vi "Test1_1b_ASIC_pepe.vi"(0 "Instrument VISA in":T1={"AWG VISA"="generadorpulsos", "Oscilloscope  VISA "="Oscilloscope", "Integration Board IP"="172.16.7.43", "connection ID"=refnum, "report out"=refnum, "report file path"=path "D:/CTA/Data_test/ASIC/test3a"}, 1 "threshold":i32[][](array[numeric]), 5 "quantity":i32=3, 7 "Cycles Burst":i32=10000, 11 "error in":errorcluster={"status"=FALSE, "code"=0, "source"="VISA Write in Test2_3a_ASIC_fast.vi->test_sum_ASIC.vi"}, 12 "channel array":i32[](array[numeric])=[0, 1, 2, 3, 4, 5, 6], 13 "Voltages comprobation":dbl[](array[numeric])=[0.05, 0.1, 0.2, 0.3, 0.4, 0.5, 0.6, 0.7, 0.8, 1.0]) -> (4 "Instrument VISA out":T1, 15 "error out":errorcluster)   [LabVIEW 2009]
uses:
  <vilib>/Utility/NIReport.llb/NI_report.lvclass
  <vilib>/Utility/NIReport.llb/HTML/NI_HTML.lvclass
  <instrlib>/Agilent 8000 Series/Public/Configure/Configure Math (Binary Operation).vi
  <instrlib>/Agilent 81150/Agilent 81150.lvlib
  L0_Asic/L0 Asic Test Folder v9/C/Program Files/National Instruments/LabVIEW 2012/instr.lib/Agilent 8000 Series/Agilent 8000 Series.lvlib
panel:
  out "read buffer 4":string="V amptd(f2),1.074E+00,0,1.056E+00,1.087E+00,1.0690E+00,5.5E-03,9.4E+01,+ width(f2),2.90015E-09,0,2.90015E-09,2.95960E-09,2.925838E-09,1.2702E-11,9.4E+01,V amptd(1),5.5E-02,0,4.8E-02,6.7E-02,5.55E-02,3.5E-03,9.4E+01,+ width(f1),9.99999E+37,5,9.99999E+37,9.99999E+37,9.99999E+37,9.99999E+37,9.99999E+37,Time(f1-f2),6.26722E-09,0,6.20145E-09,6.35270E-09,6.264189E-09,3.2805E-11,9.4E+01\n"
  out "report file path":path=path "D:/CTA/Data_test/test3a"
  out "Array":i32[](array[numeric])=[2, 3, 5]
  out "points quantity":dbl=94.0
  out "ouput data array":dbl[](array[numeric])=[0.75, 42.0, 0.0, 63.0, 1.0, 1.069, 0.0055, 2.925838e-09, 1.2702e-11, 0.0555, 0.0035, 9.99999e+37, 9.99999e+37, 6.264189e-09, 3.2805e-11, 94.0]
  out "read buffer 3":string="V amptd(f2),1.074E+00,0,1.056E+00,1.087E+00,1.0690E+00,5.5E-03,9.4E+01,+ width(f2),2.90015E-09,0,2.90015E-09,2.95960E-09,2.925838E-09,1.2702E-11,9.4E+01,V amptd(1),5.5E-02,0,4.8E-02,6.7E-02,5.55E-02,3.5E-03,9.4E+01,+ width(f1),9.99999E+37,5,9.99999E+37,9.99999E+37,9.99999E+37,9.99999E+37,9.99999E+37,Time(f1-f2),6.26722E-09,0,6.20145E-09,6.35270E-09,6.264189E-09,3.2805E-11,9.4E+01\n"
  in  "Voltage":dbl[](array[numeric])=[0.05, 0.2, 0.5, 0.7, 1.0]
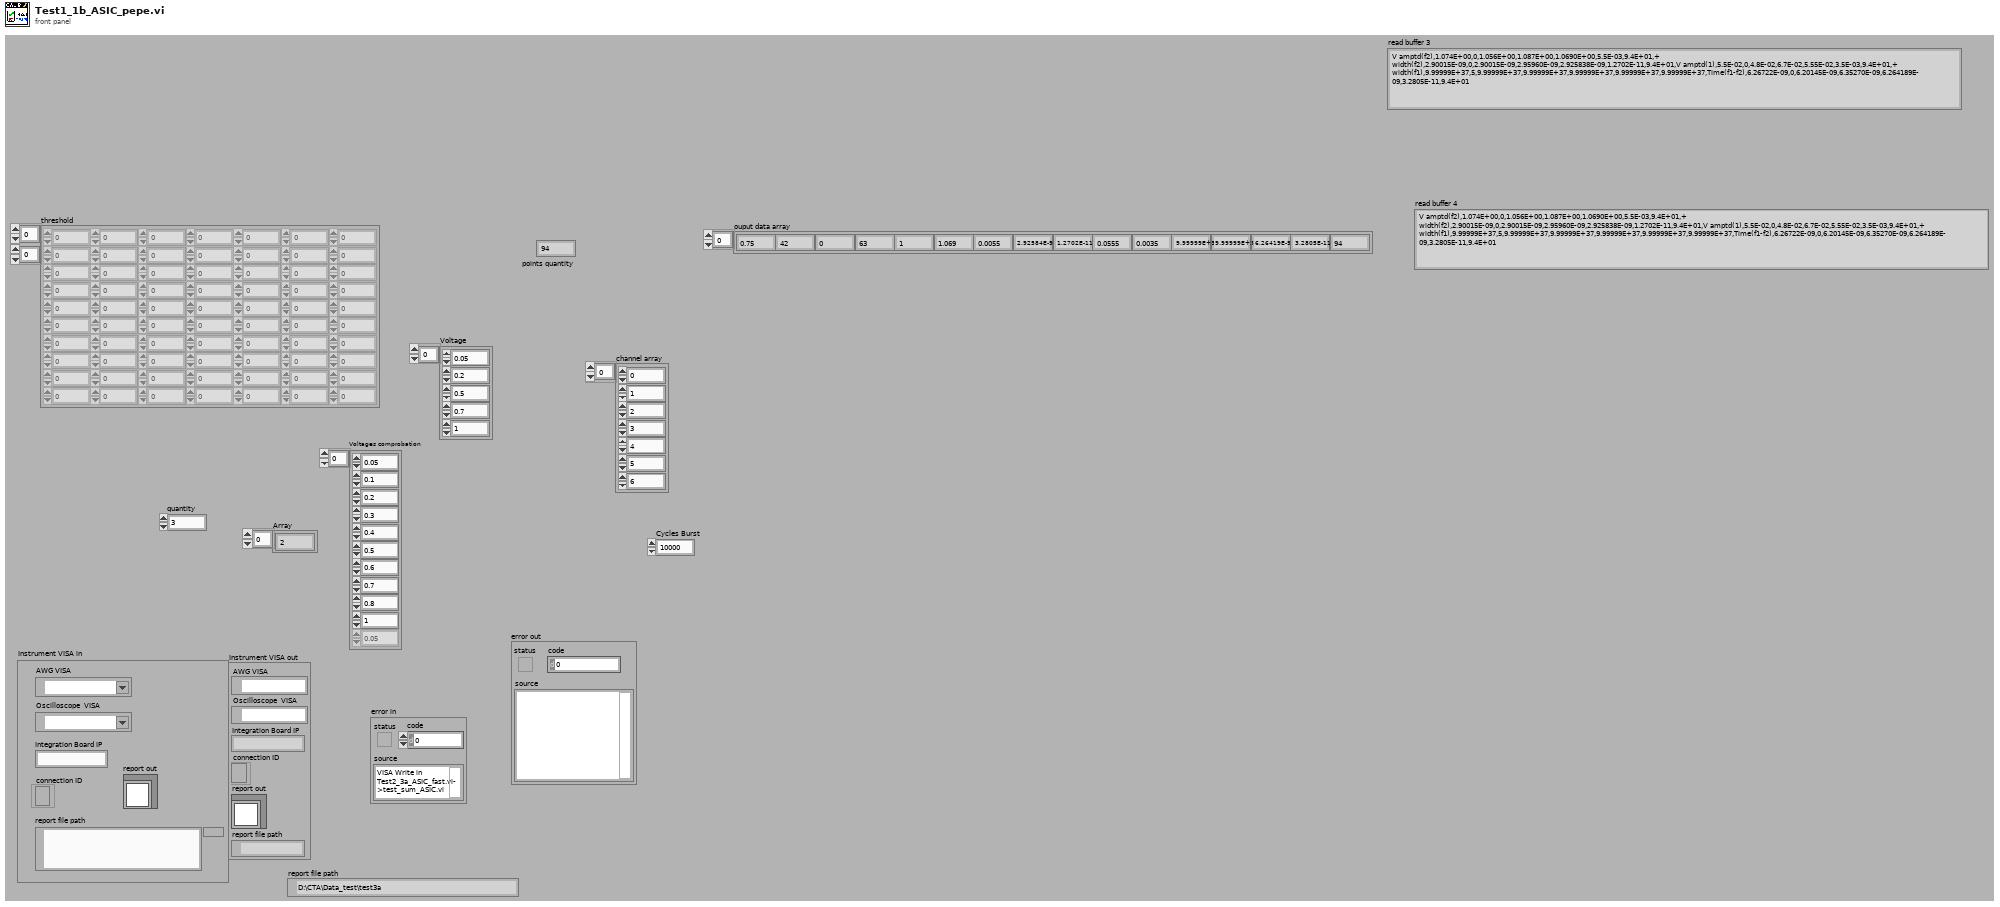
[diagram p1: front panel]
types:
  T1 = cluster{"AWG VISA":refnum<visa-resource-name>, "Oscilloscope  VISA ":refnum<visa-resource-name>, "Integration Board IP":string, "connection ID":refnum<k5>, "report out":refnum<class "NI_report.lvclass">, "report file path":path}
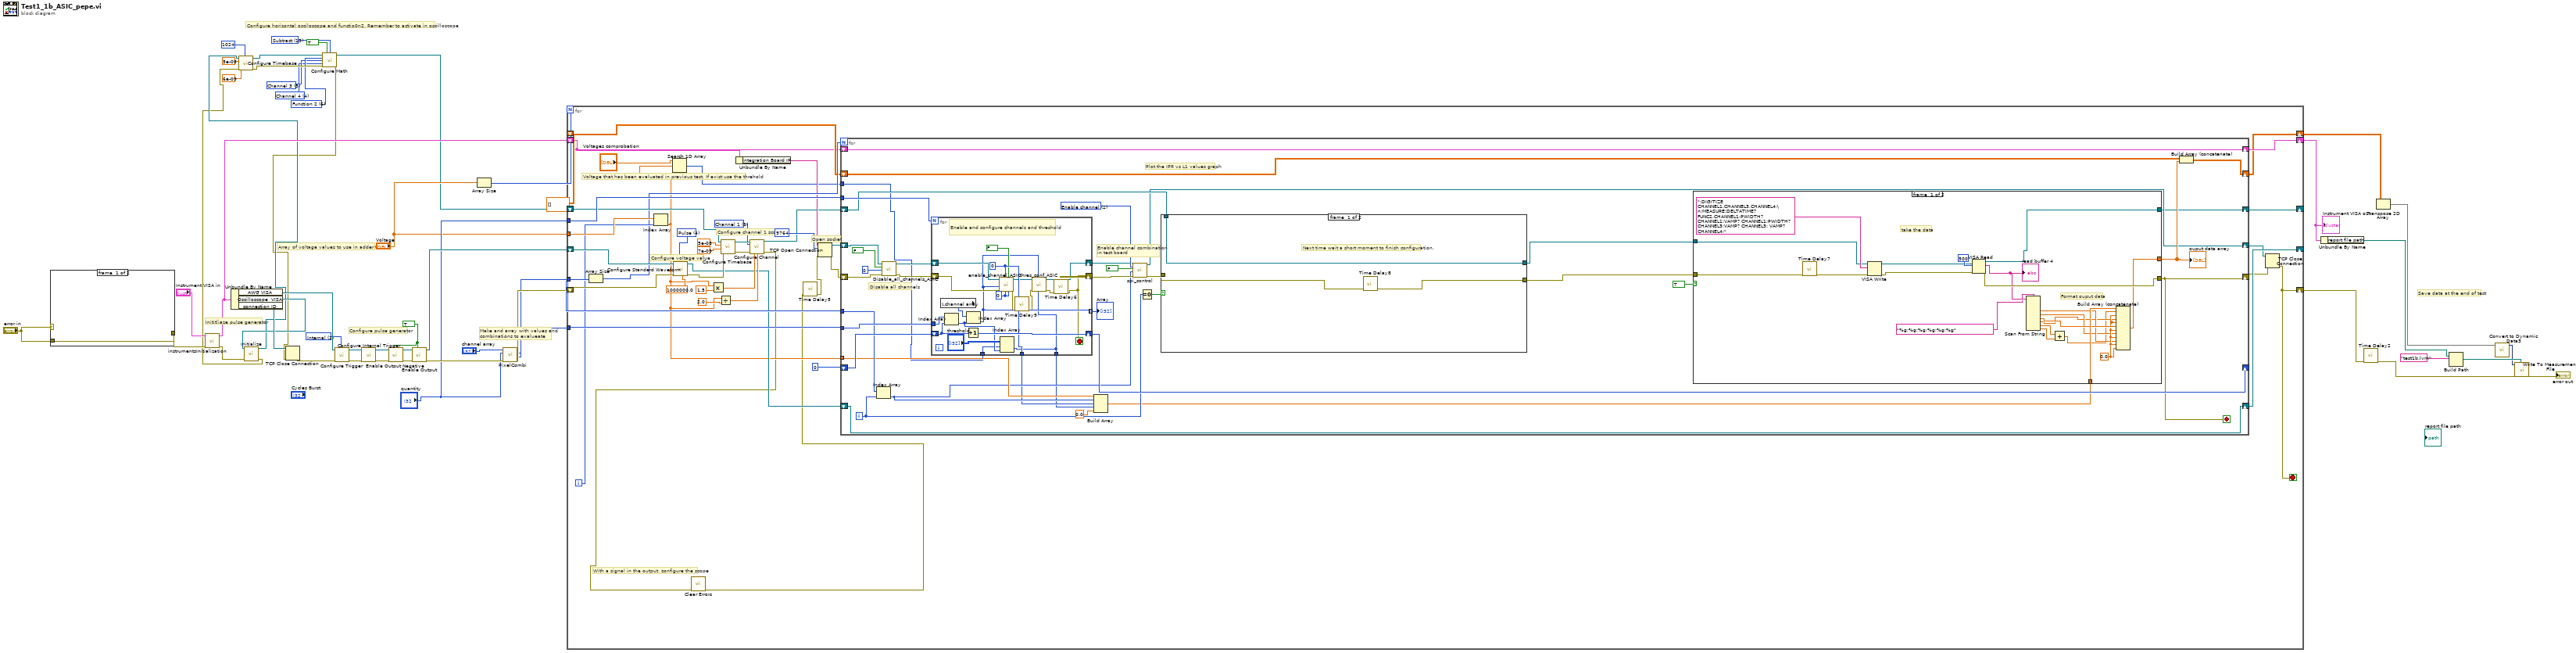
[diagram p0: block diagram]
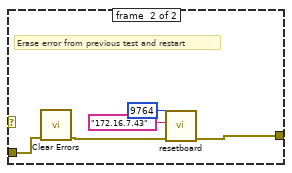
[diagram p2: hidden frame]
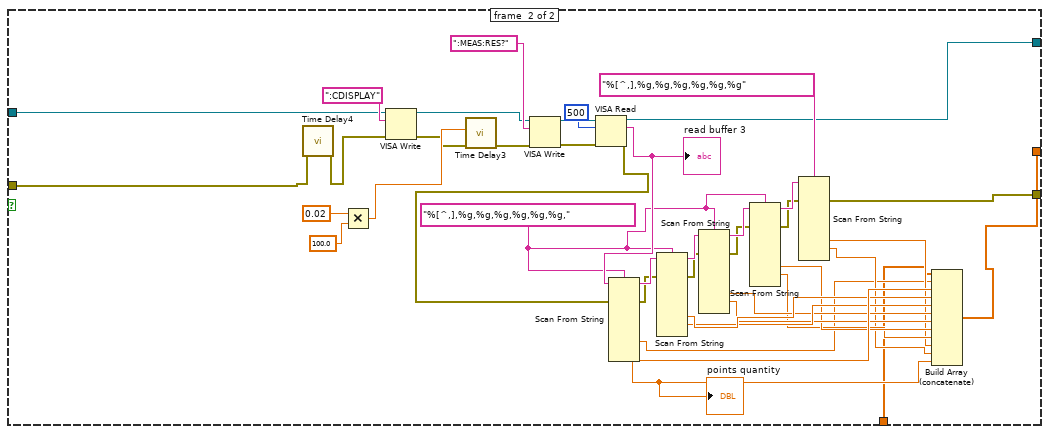
[diagram p3: hidden frame]
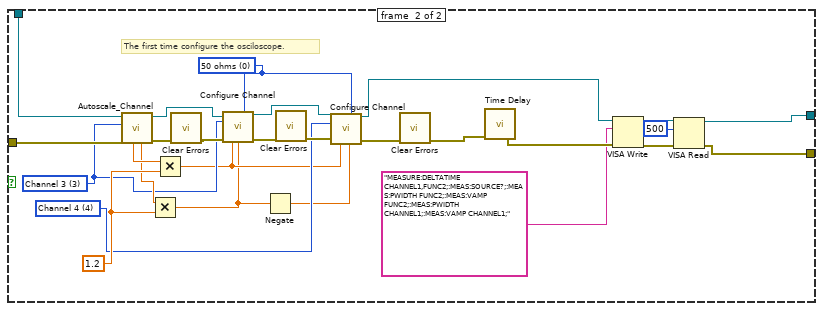
[diagram p4: hidden frame]
diagram:
  w8 = u16 6 items=["Function 1"=5, "Function 2"=6, "Function 3"=7, "Function 4"=8] ("Math Channel (5: Function 1)")
  w12 = u16 15 items=["Add"=12, "Divide"=13, "Multiply"=14, "Subtract"=15, "Common Mode"=16, "Versus"=17] ("Math Operation (12: Add)")
  w7 = 3 items=["Channel 1"=1, "Channel 2"=2, "Channel 3"=3, "Channel 4"=4] ("Channel (1: Channel 1)")
  w6 = 4 items=["Channel 1"=1, "Channel 2"=2, "Channel 3"=3, "Channel 4"=4] ("Channel (1: Channel 1)")
  w32 = u16 1 items=["Immediate", "Internal", "External", "Software Trigger Function"] ("Trigger Source (0: Immediate)")
  w19 = TRUE ("Enable Output (T: Enable)")
  # "Configure horizontal osciloscope and functio0n2. Remember to activate in oscilloscope"
  # "Save data at the end of test"
  # "Array of voltage values to use in adder test"
  # "Make and array with values and \ncombinations to evalueate"
  # "Configure pulse generator"
  # "Inititliaze pulse generator"
  n1 = case shown="No Error" "error in" {
    tunnel: "error in" -> [w52 w54]
    tunnel: [w52 w57] -> w28
    frame #0 {
    }
    frame #1 {
      # "Erase error from previous test and restart"
      n2 = call <vilib>:"Clear Errors.vi"("error in (no error)"=w54) -> ("error out"=w53:errorcluster)  [unwired: 6 in]
      n3 = call "resetboard.vi"("error in (no error)"=w53, "address"="172.16.7.43", "remote port or service name"=u16 9764) -> ("error out"=w57:errorcluster)  [unwired: 7 in, 1 out]
    }
  }
  n4 = call "instrumentsInitialization.vi"("error in"=w28, "Instrument VISA in"="Instrument VISA in") -> ("error out"=w16:errorcluster, "Instrument VISA out"=w25:T1)  [unwired: 8 in]
  n5 = Unbundle By Name(w25) -> ("AWG VISA"=w35:refnum<visa-resource-name>, "Oscilloscope  VISA"=w15:refnum<visa-resource-name>, "connection ID"=w27:refnum<k5>)
  n6 = call <instrlib>:"Initialize.vi"("error in (no error)"=w16, "VISA resource name"=w15) -> ("error out"=w2:errorcluster, "VISA resource name out"=w4:refnum<visa-resource-name>)  [unwired: 8 in]
  n7 = call <instrlib>:"Configure Timebase.vi"("Record Length (1000)"=1024, "error in (no error)"=w2, "Position (0.0 s)"=6e-09, "Timebase (0.005 s)"=5e-08, "VISA resource name"=w4) -> ("error out"=w9:errorcluster, "VISA resource name out"=w10:refnum<visa-resource-name>)  [unwired: 5 in]
  n8 = call-poly <instrlib>:"Configure Math.vi"("VISA resource name"=w10, "Enable Math Channel (T:Enable)"=TRUE, "Math Operation (12: Add)"=w12, "Math Channel (5: Function 1)"=w8, "Math Operand (1: Channel 1)"=w7, "Math Operand (2: Channel 2)"=w6, "error in (no error)"=w9) -> ("VISA resource name out"=w3:refnum<visa-resource-name>, "error out"=w1:errorcluster)  [unwired: 7 in]
  n9 = TCP Close Connection(connection ID=w27, error in (no error)=w1) -> (error out=w26:errorcluster)  [unwired: 1 in, 1 out]
  n10 = call <instrlib>:"Configure Trigger.vi"("Trigger Source (0: Immediate)"=w32, "error in (no error)"=w26, "VISA resource name"=w35) -> ("error out"=w33:errorcluster, "VISA resource name out"=w34:refnum<visa-resource-name>)  [unwired: 7 in]
  n11 = call <instrlib>:"Configure Internal Trigger.vi"("error in (no error)"=w33, "VISA resource name"=w34) -> ("error out"=w21:errorcluster, "VISA resource name out"=w22:refnum<visa-resource-name>)  [unwired: 8 in]
  n12 = call <instrlib>:"Enable Output Negative.vi"("Enable Output (T: Enable)"=w19, "error in (no error)"=w21, "VISA resource name"=w22) -> ("error out"=w20:errorcluster, "VISA resource name out"=w23:refnum<visa-resource-name>)  [unwired: 7 in]
  n13 = call <instrlib>:"Enable Output.vi"("Enable Output (T: Enable)"=w19, "error in (no error)"=w20, "VISA resource name"=w23) -> ("error out"=w51:errorcluster, "VISA resource name out"=w49:refnum<visa-resource-name>)  [unwired: 7 in]
  n14 = Array Size(array="Voltage") -> (size(s)=w42:i32)
  n15 = call "PixelCombi.vi"("error in"=w51, "quantity"="quantity", "array"="channel array") -> ("error out"=w50:errorcluster, "Channels"=w48:i32[], "Combination Array"=w47:i16[])  [unwired: 6 in]
  n16 = for {
    N: w42 -> [_]
    tunnel: w48 -> [w98]
    tunnel: w47 -> [w97]
    shift-right: [w86] -> w36
    shift-left: w50 -> [w100]
    tunnel: "Voltage" -> [w96]
    tunnel: "quantity" -> [w94]
    shift-right: [w90] -> w24
    shift-left: w25 -> [w64]
    shift-right: [w89] -> w17
    shift-left: dbl[][] [] -> [w91]
    shift-right: [w87] -> _
    shift-left: w49 -> [w99]
    shift-right: [w88] -> _
    shift-left: w3 -> [w93]
    i -> [w95]
    stop <- w86 stop-if-true
    w77 = 1 items=["Channel 1"=1, "Channel 2"=2, "Channel 3"=3, "Channel 4"=4] ("Channel (1: Channel 1)")
    w85 = u16 4 items=["Sine", "Square", "Ramp Up", "Ramp Down", "Pulse", "Noise", "DC"] ("Waveform (0: Sine)")
    # "With a signal in the output, configure the scope"
    # "Open socket"
    # "Configure channel 1 scope"
    # "Configure voltage value"
    # "Voltage that has been evaluated in previous test. If exist use the threhold"
    n17 = Array Size(array=w97) -> (size(s)=w92:i32)
    n18 = Index Array(array=w96, index=w95) -> (element=w63:dbl)
    n19 = Search 1D Array(1D array="Voltages comprobation", element=w63) -> (index of element=w61:i32)  [unwired: 1 in]
    n20 = call <instrlib>:"Configure Standard Waveform.vi"("Frequency (1000.0 Hz)"=1000000.0, "Waveform (0: Sine)"=w85, "error in (no error)"=w100, "Amplitude (1.0 Vpp)"=w63, "VISA resource name"=w99) -> ("error out"=w82:errorcluster, "VISA resource name out"=w66:refnum<visa-resource-name>)  [unwired: 5 in]
    n21 = Multiply(x=w63, y=1.5) -> (x*y=w76:dbl)
    n22 = Divide(x=w63, y=2.0) -> (x/y=w70:dbl)
    n23 = call <instrlib>:"Configure Timebase.vi"("error in (no error)"=w82, "Position (0.0 s)"=7e-09, "Timebase (0.005 s)"=5e-08, "VISA resource name"=w93) -> ("error out"=w81:errorcluster, "VISA resource name out"=w80:refnum<visa-resource-name>)  [unwired: 6 in]
    n24 = Unbundle By Name(w64) -> ("Integration Board IP"=w73:string)
    n25 = call "Configure Channel.vi"("VISA resource name"=w80, "Channel (1: Channel 1)"=w77, "error in (no error)"=w81, "Vertical Range (2.0 V)"=w76, "Vertical Offset (0.0 V)"=w70) -> ("VISA resource name out"=w58:refnum<visa-resource-name>, "error out"=w60:errorcluster)  [unwired: 9 in]
    n26 = call <vilib>:"Clear Errors.vi"("error in (no error)"=w60) -> ("error out"=w59:errorcluster)  [unwired: 6 in]
    n27 = call "Time Delay5"("error in (no error)"=w59) -> ("error out"=w65:errorcluster)  [unwired: 10 in]
    n28 = TCP Open Connection(address=w73, remote port or service name=u16 9764, error in (no error)=w65) -> (connection ID=w67:refnum<k5>, error out=w74:errorcluster)  [unwired: 2 in]
    n29 = for {
      N: w92 -> [_]
      tunnel: w97 -> [w135]
      tunnel: w98 -> [w136]
      shift-right: [w137] -> _
      shift-left: i16 0 ("element") -> [w138]
      shift-right: [w116] -> w69
      shift-left: w74 -> [w128]
      tunnel: w94 -> [w134]
      shift-right: [w129] -> w89
      shift-left: w91 -> [w130]
      shift-right: [w117] -> w68
      shift-left: w67 -> [w115]
      tunnel: w63 -> [w113]
      shift-right: [w109] -> w88
      shift-left: w58 -> [w122]
      shift-right: [w108] -> w87
      shift-left: w66 -> [w108]
      shift-right: [w103] -> w90
      shift-left: w64 -> [w103]
      tunnel: w61 -> [w101]
      i -> [w120]
      stop <- w116 stop-if-true
      w127 = u16 2 items=["Attenuation", "Clipping", "Enable channel", "Delay line", "ASIC"] ("Device")
      # "Enable channel combination \nin test board"
      # "Disable all channels"
      # "Plot the IPR vs L1 values graph"
      n30 = Index Array(array=w135, index=w120) -> (element=w112:i16)
      n31 = call "Disable_all_channels_ASIC.vi"("error in"=w128, "id_in"=0 ("Data"), "Clip_en_b"=FALSE, "connection ID"=w115) -> ("error out"=w132:errorcluster, "connection ID out"=w131:refnum<k5>)  [unwired: 5 in, 1 out]
      n32 = for {
        N: w134 -> [_]
        shift-right: [w249] -> w137
        shift-left: w138 -> [w250]
        tunnel: w136 -> [w248]
        shift-right: [w237] -> w125
        shift-left: w132 -> [w246]
        shift-right: [w240] -> w124
        shift-left: w131 -> [w245]
        tunnel: [w239] -> w114 mode=indexing
        tunnel: [w244] -> w111
        tunnel: [w238] -> w104
        tunnel: w101 -> [w233]
        stop <- w237 stop-if-true
        w242 = u32 0 ("Ib_clipVb")
        w244 = u32 0 ("Att gain")
        # "Enable and configure channels and threshold"
        n33 = local read "channel array"() -> (w247:i32[])
        n34 = Index Array(array=w248, index=w250) -> (element=w234:i32)
        n35 = Increment(x=w250) -> (x+1=w249:i16)
        n36 = Index Array(array=w247, index=w234) -> (element=w239:i32)
        n37 = call "enable_channel_ASIC.vi"("Clip_sel_b"=w242, "maj/sum"=FALSE, "Ib_clipVb"=w242, "Att gain"=w244, "error in"=w246, "Channel"=w239, "connection ID"=w245) -> ("error out"=w231:errorcluster, "connection ID out"=w241:refnum<k5>)  [unwired: 2 in, 1 out]
        n38 = Index Array(array="threshold", index (row)=w233, index (col)=w234) -> (element=w238:i32)
        n39 = call "Time Delay9"("error in (no error)"=w231) -> ("error out"=w232:errorcluster)  [unwired: 10 in]
        n40 = call "thres_conf_ASIC.vi"("threshold"=w238, "Ring"=w239, "error out 3"=w232, "connection ID"=w241) -> ("error out 2"=w236:errorcluster, "connection ID out"=w240:refnum<k5>)  [unwired: 4 in, 2 out]
        n41 = call "Time Delay6"("error in (no error)"=w236) -> ("error out"=w237:errorcluster)  [unwired: 10 in]
      }
      "Array" <- w114
      n42 = Build Array(w113, w112, w111, w104, 0.0 ("element")) -> (w110:dbl[])
      n43 = call "spi_control.vi"("connection ID"=w124, "Device"=w127, "Read/#write"=FALSE, "Data"=w112, "error out 3"=w125) -> ("connection ID out"=w117:refnum<k5>, "error out 2"=w123:errorcluster)  [unwired: 7 in, 6 out]
      n44 = Equal To 0?(x=w120) -> (x = 0?=w121:bool)
      n45 = case shown="True" w121 {
        tunnel: [w201 w210] -> w106
        tunnel: w123 -> [w202 w216]
        tunnel: w122 -> [w203 w217]
        tunnel: [w203 w219] -> w119
        frame #0 {
          # "Next time wait a short moment to finish configuration."
          n46 = call "Time Delay8"("error in (no error)"=w202) -> ("error out"=w201:errorcluster)  [unwired: 10 in]
        }
        frame #1 {
          w220 = u32 0 items=["50 ohms", "1 Mohms"] ("Input Impedance (1: 1 Mohms)")
          w208 = 3 items=["Channel 1"=1, "Channel 2"=2, "Channel 3"=3, "Channel 4"=4] ("Channel (1: Channel 1)")
          w207 = 4 items=["Channel 1"=1, "Channel 2"=2, "Channel 3"=3, "Channel 4"=4] ("Channel (1: Channel 1)")
          w213 = 1.2 ("y")
          # "The first time configure the osciloscope."
          n47 = call "Autoscale_Channel.vi"("error in"=w216, "Channel"=w208, "VISA resource name"=w217) -> ("error out"=w227:errorcluster, "VISA resource name out"=w230:refnum<visa-resource-name>, "Offset"=w209:dbl, "VerticalRange"=w224:dbl)  [unwired: 5 in]
          n48 = Multiply(x=w209, y=w213) -> (x*y=w205:dbl)
          n49 = Multiply(x=w224, y=w213) -> (x*y=w206:dbl)
          n50 = call <vilib>:"Clear Errors.vi"("error in (no error)"=w227) -> ("error out"=w228:errorcluster)  [unwired: 6 in]
          n51 = call "Configure Channel.vi"("VISA resource name"=w230, "Input Impedance (1: 1 Mohms)"=w220, "Channel (1: Channel 1)"=w208, "error in (no error)"=w228, "Vertical Range (2.0 V)"=w206, "Vertical Offset (0.0 V)"=w205) -> ("VISA resource name out"=w225:refnum<visa-resource-name>, "error out"=w229:errorcluster)  [unwired: 8 in]
          n52 = Negate(x=w205) -> (-x=w204:dbl)
          n53 = call <vilib>:"Clear Errors.vi"("error in (no error)"=w229) -> ("error out"=w218:errorcluster)  [unwired: 6 in]
          n54 = call "Configure Channel.vi"("VISA resource name"=w225, "Input Impedance (1: 1 Mohms)"=w220, "Channel (1: Channel 1)"=w207, "error in (no error)"=w218, "Vertical Range (2.0 V)"=w206, "Vertical Offset (0.0 V)"=w204) -> ("VISA resource name out"=w214:refnum<visa-resource-name>, "error out"=w226:errorcluster)  [unwired: 8 in]
          n55 = call <vilib>:"Clear Errors.vi"("error in (no error)"=w226) -> ("error out"=w215:errorcluster)  [unwired: 6 in]
          n56 = call "Time Delay"("error in (no error)"=w215) -> ("error out"=w212:errorcluster)  [unwired: 10 in]
          n57 = VISA Write(VISA resource name=w214, write buffer="MEASURE:DELTATIME CHANNEL1,FUNC2;:MEAS:SOURCE?;:MEAS:PWIDTH FUNC2;:MEAS:VAMP FUNC2;:MEAS:PWIDTH CHANNEL1;:MEAS:VAMP CHANNEL1;", error in (no error)=w212) -> (VISA resource name out=w223:refnum<visa-resource-name>, error out=w222:errorcluster)  [unwired: 1 out]
          n58 = VISA Read(VISA resource name=w223, byte count=u32 500, error in (no error)=w222) -> (VISA resource name out=w219:refnum<visa-resource-name>, error out=w210:errorcluster)  [unwired: 2 out]
        }
      }
      n59 = case shown="True" TRUE {
        tunnel: w119 -> [w156 w168]
        tunnel: [w151 w166] -> w118
        tunnel: [w154 w165] -> w116
        tunnel: w110 -> [w152 w163]
        tunnel: [w153 w162] -> w109
        tunnel: w106 -> [w155 w160]
        frame #0 {
          w147 = 0.0 ("output 7")
          # "Format ouput data"
          # "take the data"
          n60 = call "Time Delay7"("error in (no error)"=w155) -> ("error out"=w157:errorcluster)  [unwired: 10 in]
          n61 = VISA Write(VISA resource name=w156, write buffer=":DIGITIZE CHANNEL1,CHANNEL3,CHANNEL4;\n:MEASURE:DELTATIME? FUNC2,CHANNEL1;PWIDTH? CHANNEL1;VAMP? CHANNEL1;PWIDTH? CHANNEL3;VAMP? CHANNEL3; VAMP? CHANNEL4;", error in (no error)=w157) -> (VISA resource name out=w150:refnum<visa-resource-name>, error out=w149:errorcluster)  [unwired: 1 out]
          n62 = VISA Read(VISA resource name=w150, byte count=u32 500, error in (no error)=w149) -> (VISA resource name out=w153:refnum<visa-resource-name>, read buffer=w146:string, error out=w154:errorcluster)  [unwired: 1 out]
          "read buffer 4" <- w146
          n63 = Scan From String(format string="%g;%g;%g;%g;%g;%g", input string=w146) -> (output 1=w144:dbl, output 2=w143:dbl, output 3=w148:dbl, output 4=w142:dbl, output 5=w141:dbl, output 6=w140:dbl)  [unwired: 8 in, 3 out]
          n64 = Add(x=w141, y=w140) -> (x+y=w139:dbl)
          n65 = Build Array (concatenate)(w152, w139, w147, w142, w147, w148, w147, w143, w147, w144, w147, w147) -> (w151:dbl[])
        }
        frame #1 {
          w186 = "%[^,],%g,%g,%g,%g,%g,%g," ("format string")
          n66 = call "Time Delay4"("error in (no error)"=w160) -> ("error out"=w161:errorcluster)  [unwired: 10 in]
          n67 = Multiply(x=0.02, y=100.0) -> (x*y=w193:dbl)
          n68 = VISA Write(VISA resource name=w168, write buffer=":CDISPLAY", error in (no error)=w161) -> (VISA resource name out=w171:refnum<visa-resource-name>, error out=w169:errorcluster)  [unwired: 1 out]
          n69 = call "Time Delay3"("error in (no error)"=w169, "Delay Time (s)"=w193) -> ("error out"=w192:errorcluster)  [unwired: 9 in]
          n70 = VISA Write(VISA resource name=w171, write buffer=":MEAS:RES?", error in (no error)=w192) -> (VISA resource name out=w200:refnum<visa-resource-name>, error out=w199:errorcluster)  [unwired: 1 out]
          n71 = VISA Read(VISA resource name=w200, byte count=u32 500, error in (no error)=w199) -> (VISA resource name out=w162:refnum<visa-resource-name>, read buffer=w196:string, error out=w176:errorcluster)  [unwired: 1 out]
          "read buffer 3" <- w196
          n72 = Scan From String(format string=w186, input string=w196, error in=w176) -> (remaining string=w190:string, error out=w172:errorcluster, output 5=w164:dbl, output 6=w191:dbl, output 7=w177:dbl)  [unwired: 12 in, 1 out]
          "points quantity" <- w177
          n73 = Scan From String(format string=w186, input string=w190, error in=w172) -> (remaining string=w187:string, error out=w173:errorcluster, output 5=w184:dbl, output 6=w183:dbl)  [unwired: 13 in, 1 out]
          n74 = Scan From String(format string=w186, input string=w187, error in=w173) -> (remaining string=w188:string, error out=w174:errorcluster, output 5=w182:dbl, output 6=w181:dbl)  [unwired: 13 in, 1 out]
          n75 = Scan From String(format string=w186, input string=w188, error in=w174) -> (remaining string=w189:string, error out=w175:errorcluster, output 5=w180:dbl, output 6=w179:dbl)  [unwired: 13 in, 1 out]
          n76 = Scan From String(format string="%[^,],%g,%g,%g,%g,%g,%g", input string=w189, error in=w175) -> (error out=w165:errorcluster, output 5=w167:dbl, output 6=w178:dbl)  [unwired: 13 in, 2 out]
          n77 = Build Array (concatenate)(w163, w164, w191, w184, w183, w182, w181, w180, w179, w167, w178, w177) -> (w166:dbl[])
        }
      }
      "ouput data array" <- w118
      n78 = Build Array (concatenate)(w130, w118) -> (w129:dbl[][])
    }
    n79 = TCP Close Connection(connection ID=w68, error in (no error)=w69) -> (error out=w86:errorcluster)  [unwired: 1 in, 1 out]
  }
  "Instrument VISA out" <- w24
  n80 = Unbundle By Name(w24) -> ("report file path"=w45:path)
  n81 = call "Time Delay2"("error in (no error)"=w36) -> ("error out"=w43:errorcluster)  [unwired: 10 in]
  n82 = Transpose 2D Array(2D array=w17) -> (transposed array=w30:dbl[][])
  n83 = Build Path(base path=w45, name or relative path="test1b.lvm" ("string")) -> (appended path=w44:path)
  n84 = call "Convert to Dynamic Data3"("2D Array"=w30) -> ("Dynamic Data Type"=w31:dynamicdata)  [unwired: 3 in]
  n85 = call "Write To Measurement File"("Signals"=w31, "error in (no error)"=w43, "Filename"=w44) -> ("error out"=→"error out":errorcluster)  [unwired: 14 in, 2 out]
